vi "Read App Configuration Path.vi"(9 "PythonConfiguration in":refnum<class "PythonConfiguration.lvclass">) -> (3 "PythonConfiguration out":refnum<class "PythonConfiguration.lvclass">, 4 "App Configuration Path":path)   [LabVIEW 2014, in "Raspberry Pi Compatible Compiler for LabVIEW.lvlib" / "PythonConfiguration.lvclass"]
uses:
  PythonConfiguration.lvclass
  PythonConfiguration.lvclass/PythonConfiguration.ctl
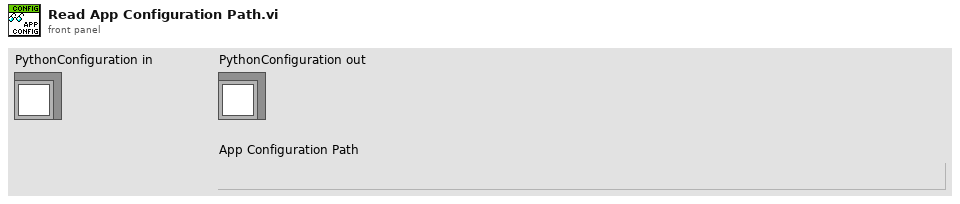
[diagram p1: front panel]
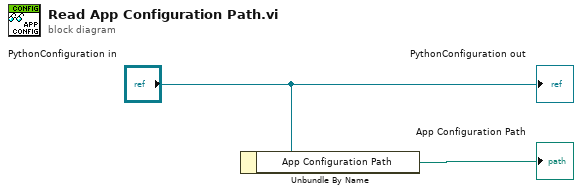
[diagram p0: block diagram]
diagram:
  n1 = Unbundle By Name("PythonConfiguration in") -> ("App Configuration Path"=→"App Configuration Path":path)
  "PythonConfiguration out" <- "PythonConfiguration in"
